vi "gxml_SearchParser.vi"(8 "error in":errorcluster, 9 "TypeDesc":variant, 10 "XML String In":string) -> (0 "error out":errorcluster, 2 "Parsed Data":variant)   [LabVIEW 2011, in "Third Party VIs.lvlib" / "GXML.lvlib"]
doc: "Using a custom XML schema, this VI converts an XML string into a user specified LabVIEW data type. The data structure is defined by the input <b>TypeDesc</b> and its elements must have the same name and hierarchy as the elements in the XML string.\n\nThis VI employs a recursive searching algorithm so the order of the elements is not important, only their hierarchy. Furthermore since this VI recursively searches for XML content by name, the XML file is allowed to have extra items not referenced by the type definition."
uses:
  GXML.lvlib
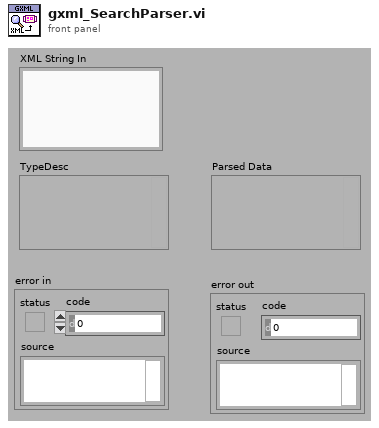
[diagram p1: front panel]
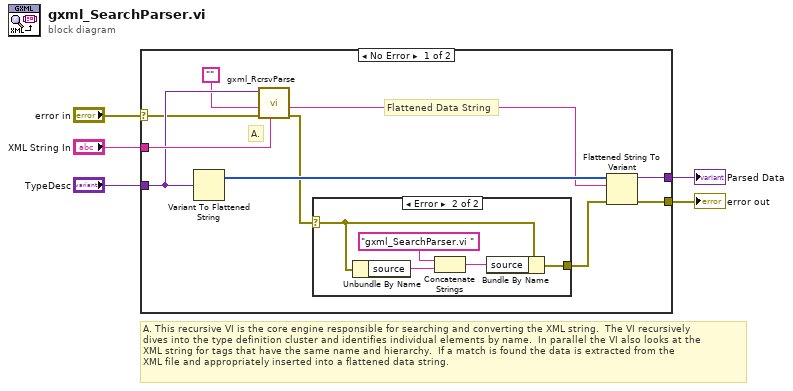
[diagram p0: block diagram]
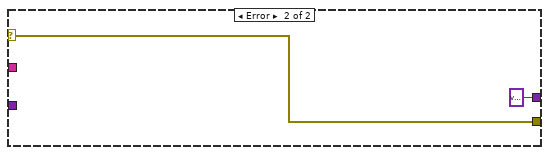
[diagram p3: hidden frame]
diagram:
  # "A. This recursive VI is the core engine responsible for searching and converting the XML string.  The VI recursively \ndives into the type definition cluster and identifies individual elements by name.  In parallel the VI also looks at the \nXML string for tags that have the same name and hierarchy.  If a match is found the data is extracted from the \nXML file and appropriately inserted into a flattened data string."
  n1 = case shown="No Error" "error in" {
    selector: "error in" -> [w7 w23]
    tunnel: [w14 variant ("Variant")] -> w5
    tunnel: "XML String In" -> [w13 _]
    tunnel: "TypeDesc" -> [w12 _]
    tunnel: [w8 w23] -> w2
    frame No Error {
      # "Flattened Data String"
      # "A."
      n2 = Variant To Flattened String(Variant=w12) -> (1:w15:i16[])  [unwired: 1 out]
      n3 = call "gxml_RcrsvParse.vi"("File Item Contents"=w13, "error in"=w7, "Flat String In"="", "Item TypeDesc"=w12) -> ("error out"=w10:errorcluster, "Flat String Out"=w11:string)  [unwired: 6 in]
      n4 = case shown="Error" w10 {
        selector: w10 -> [w16 w18]
        tunnel: [w16 w17] -> w9
        frame No Error {
        }
        frame Error {
          n5 = Unbundle By Name(w18) -> ("source"=w21:string)
          n6 = Concatenate Strings("gxml_SearchParser.vi ", w21) -> (w19:string)
          n7 = Bundle By Name(cluster=w18, "source"=w19) -> (w17:errorcluster)
        }
      }
      n8 = Flattened String To Variant(4:w9, 6:w11, 7:w15) -> (0:w8:errorcluster, 3:w14:variant)
    }
    frame Error {
    }
  }
  "error out" <- w2
  "Parsed Data" <- w5
